vi "Actor Core.vi"(8 "error in":errorcluster, 11 "ConfigurationLayout in":refnum<class "LeftListboxViewManager.lvclass">=refnum) -> (0 "error out":errorcluster, 3 "Actor out":refnum<class "Actor.lvclass">)   [LabVIEW 2020, in "LeftListboxViewManager.lvlib" / "LeftListboxViewManager.lvclass"]
doc: "(<B>Filename</B>: Actor Framework.lvlib:Actor.lvclass:Actor Core.vi)\n\nReceives messages to the actor, reacts to them, and initiates any error handling that may shut the actor down.\n\nDescendant classes may override this VI to append parallel tasks for the actor to complete while it handles messages. Overrides use the Call Parent Method node.\n\n<License>\nCopyright © 2017 Composed Systems, LLC | All rights reserved\nwww.composed.io\n\nAuthor: Ethan Stern <ethan.stern@composed.io>\n\nThis software is provided \"AS IS\" WITHOUT WARRANTIES, either express or implied, AND IS FOR EDUCATIONAL PURPOSES ONLY.\n</License>"
uses:
  <vilib>/gpm_packages/@cs/ViewManager/source/LeftListboxViewManager/LeftListboxViewManager.lvclass
  C:/Program Files/National Instruments/LabVIEW 2020/vi.lib/gpm_packages/@cs/mva-viewable/Source/IViewManager/IViewManager/IViewManager.lvclass
  C:/Program Files/National Instruments/LabVIEW 2020/vi.lib/ActorFramework/Actor/Actor.lvclass
  <vilib>/ActorFramework/Actor/Actor.lvclass
  <vilib>/gpm_packages/@cs/ViewManager/source/LeftListboxViewManager/LeftListboxViewManager.lvclass/LeftListboxViewManager.ctl
  <vilib>/ActorFramework/Actor/Actor.lvclass/Actor.ctl
  <vilib>/ActorFramework/Message Enqueuer/Message Enqueuer.lvclass/Message Enqueuer.ctl
  <vilib>/gpm_packages/@cs/ViewManager/source/LeftListboxViewManager Messages/Set View by Listbox Index Msg/Set View by Listbox Index Msg.lvclass/Set View by Listbox Index Msg.ctl
  <vilib>/ActorFramework/Message Enqueuer/Init from Existing Queue.vi
  <vilib>/ActorFramework/Message Enqueuer/Enqueue.vi
  <vilib>/gpm_packages/@cs/ViewManager/source/LeftListboxViewManager Messages/Set View by Listbox Index Msg/Set View by Listbox Index Msg.lvclass
  C:/Program Files/National Instruments/LabVIEW 2020/vi.lib/ActorFramework/Message/Message.lvclass
  <vilib>/ActorFramework/Message Priority Queue/Priority Enqueue.vi
  <vilib>/ActorFramework/Message Enqueuer/Message Enqueuer.lvclass
  <vilib>/gpm_packages/@cs/mva-viewable/Source/IViewManager/IViewManager/IViewManager.lvclass
  <vilib>/gpm_packages/@cs/mva-viewable/Source/IViewable/ProtectedSubpanel/ProtectedSubpanel.lvclass
panel:
  in  "Listbox":i32(listbox)
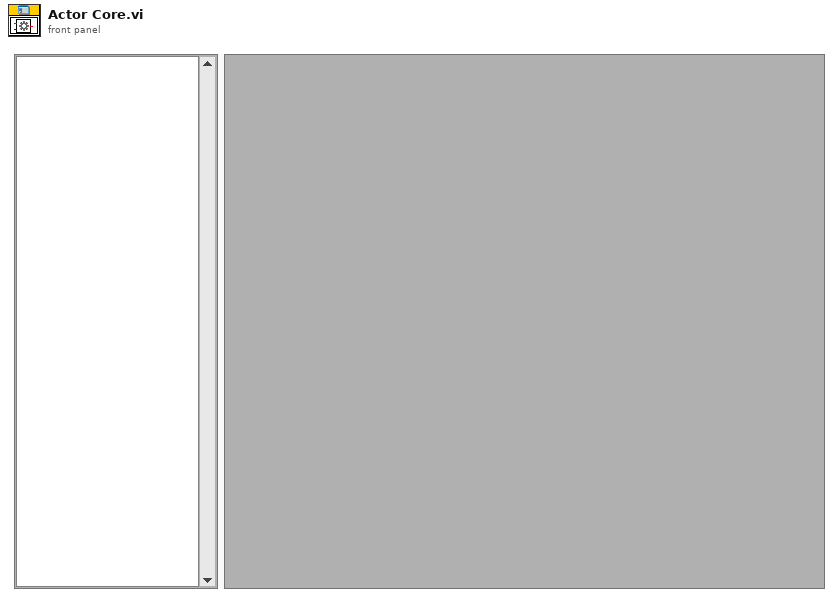
[diagram p1: front panel]
types:
  T1 = typedef "IViewable.lvlib/ProtectedSubpanel.lvclass/Protected Subpanel Reference.ctl" = refnum<data-value>
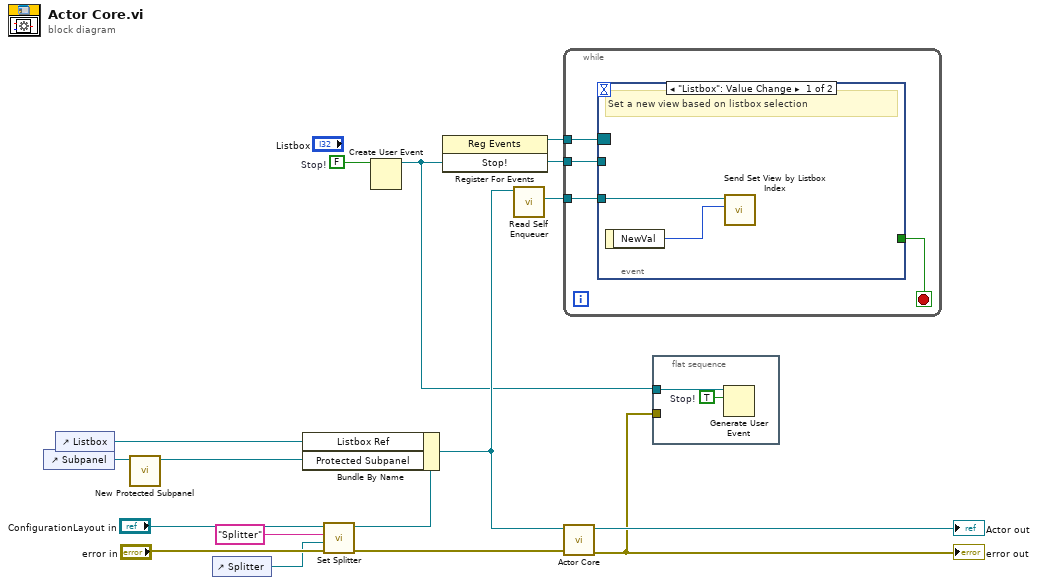
[diagram p0: block diagram]
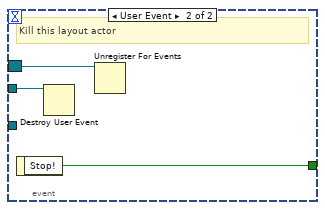
[diagram p2: hidden frame]
diagram:
  w12 = FALSE  # Stop!
  n1 = control-ref of="Subpanel"() -> (w7:refnum<vi>)
  n2 = control-ref of="Listbox"() -> (w15:refnum<vi>)
  n3 = call <vilib>:"New Protected Subpanel.vi"("SubPnl Refnum"=w7) -> ("Protected Subpanel"=w8:T1)  [unwired: 9 in, 1 out]
  n4 = control-ref of="Splitter"() -> (w2:refnum<vi>)
  n5 = call <vilib>:"Set Splitter.vi"("error in (no error)"="error in", "Splitter Reference"=w2, "Splitter Name"="Splitter", "IViewManager in"="ConfigurationLayout in") -> ("error out"=w4:errorcluster, "IViewManager out"=w3:refnum<class "LeftListboxViewManager.lvclass">)  [unwired: 6 in]
  n6 = Bundle By Name(cluster=w3, "Listbox Ref"=w15, "Protected Subpanel"=w8) -> (w14:refnum<class "LeftListboxViewManager.lvclass">)
  n7 = Create User Event(user event datatype=w12) -> (user event=w10:refnum<user-event>)  [unwired: 1 in, 1 out]
  n8 = register-events(w10) -> (reference out=w11:refnum<event-registration>)  [unwired: 2 in, 1 out]
  n9 = call <vilib>:"Read Self Enqueuer.vi"("Actor"=w14) -> ("Self Enqueuer"=w13:refnum<class "Message Enqueuer.lvclass">)  [unwired: 10 in]
  n10 = while {
    tunnel: w13 -> [w20]
    tunnel: w11 -> [w19]
    tunnel: w10 -> [w17]
    stop <- w18 stop-if-true
    n11 = event shown="[0] \"Listbox\": Value Change" {
      selector: w19 -> [_ w24]
      dyn-events: _ -> [_ _]
      timeout: _ -> [_ _]
      tunnel: w20 -> [w22 _]
      tunnel: [_ w25] -> w18
      tunnel: w17 -> [_ w23]
      event "Listbox": Value Change {
        # "Set a new view based on listbox selection"
        n12 = event-data() -> ("NewVal"=w21:i32)  [unwired: 1 in]
        n13 = call <vilib>:"Send Set View by Listbox Index.vi"("Index"=w21, "Message Enqueuer"=w22) -> ()  [unwired: 8 in, 2 out]
      }
      event User Event {
        # "Kill this layout actor"
        n14 = event-data() -> ("Stop!"=w25:bool)  [unwired: 1 in]
        n15 = Destroy User Event(user event=w23) -> ()  [unwired: 1 in, 1 out]
        n16 = Unregister For Events(event registration refnum=w24) -> ()  [unwired: 1 in, 1 out]
      }
    }
  }
  n17 = call-parent "Actor Core.vi"("error in"=w4, "IViewable In"=w14) -> ("error out"=w9:errorcluster, "Actor out"=→"Actor out":refnum<class "Actor.lvclass">)  [unwired: 8 in]
  "error out" <- w9
  n18 = flat-sequence {
    tunnel: w10 -> [w26]
    tunnel: w9 -> [_]
    frame #0 {
      w27 = TRUE  # Stop!
      n19 = Generate User Event(user event=w26, event data cluster=w27) -> ()  [unwired: 2 in, 2 out]
    }
  }
